vi "2D Guassian - Fit Image U16.vi"(7 "Image In (U16)":u16[][](array[numeric])) -> (8 "Best Fit Params":T1)   [LabVIEW 2016]
uses:
  2D Gaussian - Type Defs/2D Gaussian - Best Fit Parameters.ctl
  <vilib>/gmath/NumericalOptimization/Nonlinear Curve Fit LM bound.vi
  <vilib>/gmath/NI_Gmath.lvlib
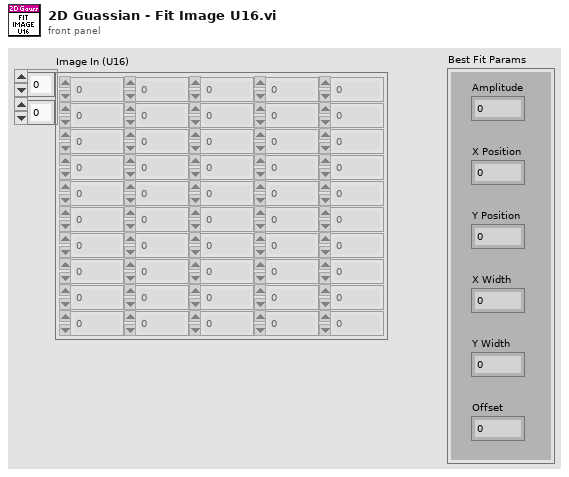
[diagram p1: front panel]
types:
  T1 = typedef "2D Gaussian - Best Fit Parameters.ctl" = cluster{"Amplitude":dbl, "X Position":dbl, "Y Position":dbl, "X Width":dbl, "Y Width":dbl, "Offset":dbl}
  T2 = cluster{"parameter minimum":dbl[], "parameter maximum":dbl[]}
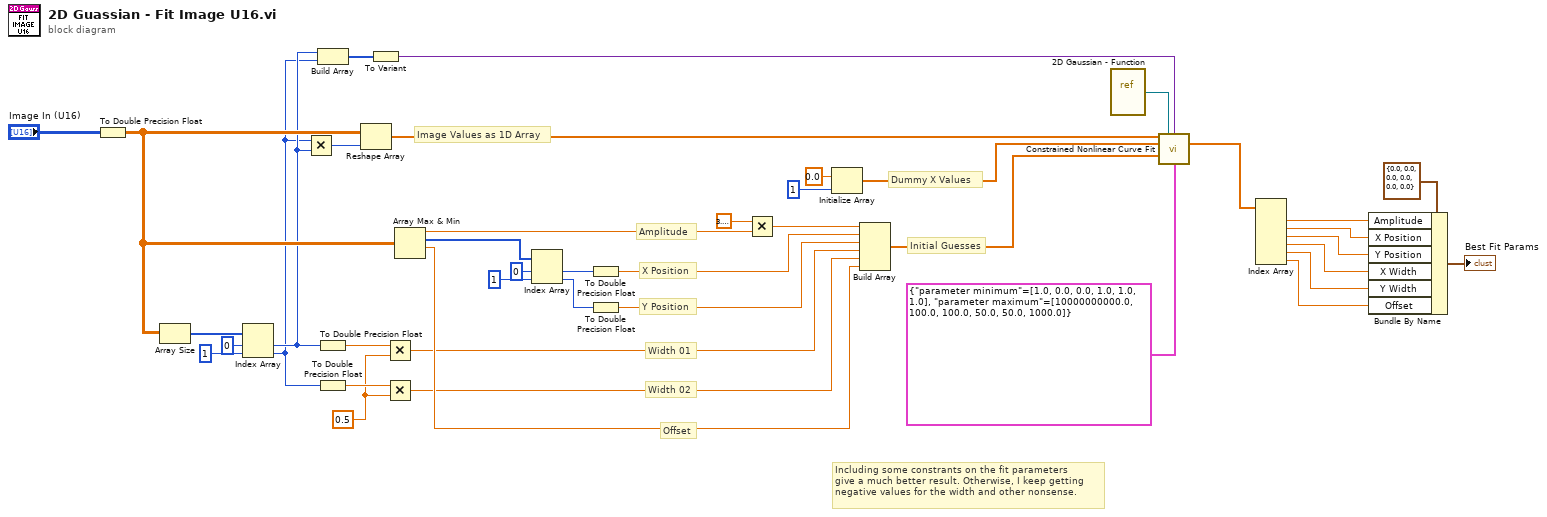
[diagram p0: block diagram]
diagram:
  w24 = 0.5
  # "Including some constrants on the fit parameters\ngive a much better result. Otherwise, I keep getting\nnegative values for the width and other nonsense."
  # "Dummy X Values"
  # "Image Values as 1D Array"
  # "Initial Guesses"
  # "Width 02"
  # "Width 01"
  # "Y Position"
  # "X Position"
  # "Offset"
  # "Amplitude"
  n1 = To Double Precision Float(number="Image In (U16)") -> (double precision float=w17:dbl[][])
  n2 = Array Size(array=w17) -> (size(s)=w27:i32[])
  n3 = Index Array(array=w27, index #1=0 ("index"), index #2=1 ("index")) -> (element #1=w14:i32, element #2=w13:i32)
  n4 = Multiply(x=w13, y=w14) -> (x*y=w20:i32)
  n5 = Build Array(w14, w13) -> (w12:i32[])
  n6 = To Double Precision Float(number=w14) -> (double precision float=w26:dbl)
  n7 = To Double Precision Float(number=w13) -> (double precision float=w25:dbl)
  n8 = Reshape Array(w17, w20) -> (w21:dbl[])
  n9 = To Variant(anything=w12) -> (Variant=w11:variant)
  n10 = Multiply(x=w26, y=w24) -> (x*y=w23:dbl)
  n11 = Multiply(x=w25, y=w24) -> (x*y=w22:dbl)
  n12 = Array Max & Min(array=w17) -> (max value=w39:dbl, max index (indices)=w36:i32[], min value=w37:dbl)  [unwired: 1 out]
  n13 = Index Array(array=w36, index #1=0 ("index"), index #2=1 ("index")) -> (element #1=w33:i32, element #2=w31:i32)
  n14 = To Double Precision Float(number=w33) -> (double precision float=w32:dbl)
  n15 = To Double Precision Float(number=w31) -> (double precision float=w30:dbl)
  n16 = Multiply(x=3.141592653589793, y=w39) -> (x*y=w38:dbl)
  n17 = Initialize Array(0.0 ("element"), 1 ("dimension size")) -> (w18:dbl[])
  n18 = Build Array(w38, w32, w30, w23, w22, w37) -> (w16:dbl[])
  n19 = vi-ref "2D Gaussian - Function.vi"() -> (w42:refnum<vi>)
  n20 = call-poly <vilib>:"Constrained Nonlinear Curve Fit.vi"("Y"=w21, "f(x,a)"=w42, "data"=w11, "X"=w18, "initial parameters"=w16, "parameter bounds"=T2 {"parameter minimum"=[1.0, 0.0, 0.0, 1.0, 1.0, 1.0], "parameter maximum"=[10000000000.0, 100.0, 100.0, 50.0, 50.0, 1000.0]}) -> ("best fit parameters"=w9:dbl[])  [unwired: 4 in, 5 out]
  n21 = Index Array(array=w9) -> (element #1=w8:dbl, element #2=w7:dbl, element #3=w6:dbl, element #4=w5:dbl, element #5=w4:dbl, element #6=w3:dbl)  [unwired: 6 in]
  n22 = Bundle By Name(cluster=T1 {"Amplitude"=0.0, "X Position"=0.0, "Y Position"=0.0, "X Width"=0.0, "Y Width"=0.0, "Offset"=0.0} ("Best Fit Parameters"), "Amplitude"=w8, "X Position"=w7, "Y Position"=w6, "X Width"=w5, "Y Width"=w4, "Offset"=w3) -> (→"Best Fit Params":T1)
